vi "Apend Test Suite Result to Suites Element.vi"(8 "error in (no error)":errorcluster, 9 "Test Suite Result":T1, 10 "Test Suites Element in":refnum<k20>, 11 "XML Report In":refnum<class "XML Report.lvclass">) -> (0 "error out":errorcluster, 1 "Test Suite Element":refnum<k20>, 2 "Test Suites Element out":refnum<k20>, 3 "XML Report Out":refnum<class "XML Report.lvclass">)   [LabVIEW 2020, in "XML Report.lvclass"]
uses:
  XML Report.lvclass
  Result Types/Suite Results/Test Suite Result type.ctl
  Result Types/Assertion Result/Public/TypeDefs/Status.ctl
  Result Types/Case Result/Test Case Result type.ctl
  Result Types/Method Result/Method Result type.ctl
  Result Types/Assertion Result/Assertion Result type.ctl
  Result Types/Assertion Result/Public/TypeDefs/Assertion Type.ctl
  XML Report.lvclass/XML Report.ctl
  Result Types/Suite Results/Public/Count by Status.vi
  Result Types/Case Result/Public/Read Status.vi
  Result Types/Case Result/Private/Merge Status.vi
  Result Types/Method Result/Public/Read Status.vi
  <resource>/objmgr/DOMUserDefRef.rc
  Result Types/Suite Results/Test Suite Result.lvlib
  Result Types/Assertion Result/Assertion Result.lvlib
  Result Types/Method Result/Method Result.lvlib
  Result Types/Case Result/Test Case Result.lvlib
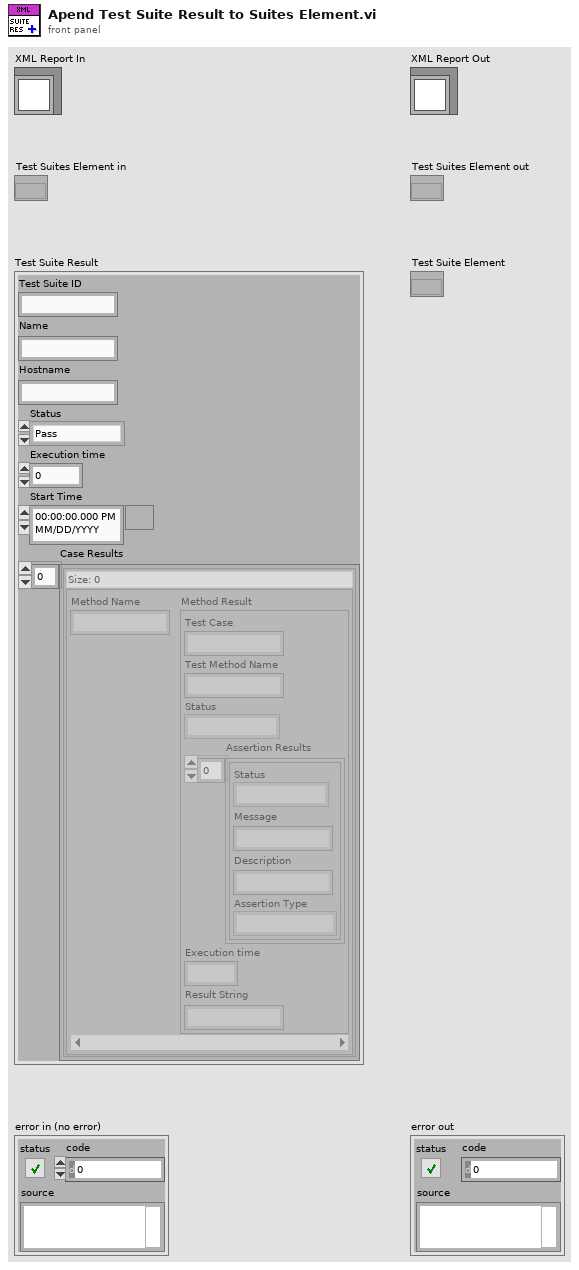
[diagram p1: front panel]
types:
  T1 = typedef "Test Suite Result.lvlib/Test Suite Result type.ctl" = cluster{"Test Suite ID":string, "Name":string, "Hostname":string, "Status":T2, "Execution time":dbl, "Start Time":timestamp, "Case Results":T3[]}
  T2 = typedef "Assertion Result.lvlib/Status.ctl" = enum16{"Pass", "Fail", "Error", "Skipped", "Setup Error", "Broken", "Teardown Error"}
  T3 = typedef "Test Case Result.lvlib/Test Case Result type.ctl" = map{string, T4}
  T4 = typedef "Method Result.lvlib/Method Result type.ctl" = cluster{"Test Case":string, "Test Method Name":string, "Status":T2, "Assertion Results":T5[], "Execution time":dbl, "Result String":string}
  T5 = typedef "Assertion Result.lvlib/Assertion Result type.ctl" = cluster{"Status":T2, "Message":string, "Description":string, "Assertion Type":T6}
  T6 = typedef "Assertion Result.lvlib/Assertion Type.ctl" = enum16{"None", "Pass", "Fail", "Skip", "Pass if Equal", "Fail if Equal", "Pass if Error", "Fail if Error", "Pass if", "Fail if"}
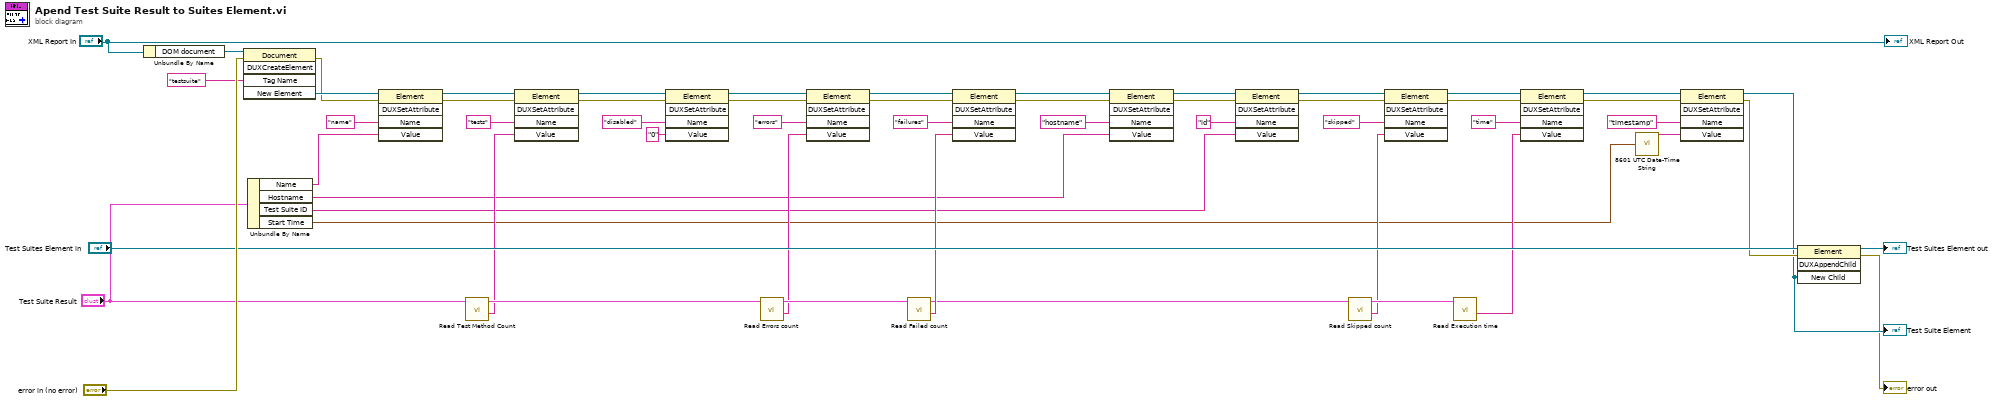
[diagram p0: block diagram]
diagram:
  n1 = Unbundle By Name("XML Report In") -> ("DOM document"=w53:refnum<k20>)
  n2 = invoke class="Document" method="DUXCreateElement"(reference=w53, error in="error in (no error)", "Tag Name"="testsuite") -> (error out=w16:errorcluster, "New Element"=w48:refnum<k20>)  [unwired: 2 in, 3 out]
  n3 = Unbundle By Name("Test Suite Result") -> ("Name"=w12:string, "Hostname"=w5:string, "Test Suite ID"=w4:string, "Start Time"=w2:timestamp)
  n4 = invoke class="Element" method="DUXSetAttribute"(reference=w48, error in=w16, "Name"="name", "Value"=w12) -> (reference out=w34:refnum<k20>, error out=w33:errorcluster)  [unwired: 1 in, 3 out]
  n5 = call "Read Test Method Count.vi"("Test Suite Result In"="Test Suite Result") -> ("Test Method count string"=w11:string, "Test Suite Result Out"=w37:T1)  [unwired: 8 in, 1 out]
  n6 = invoke class="Element" method="DUXSetAttribute"(reference=w34, error in=w33, "Name"="tests", "Value"=w11) -> (reference out=w32:refnum<k20>, error out=w31:errorcluster)  [unwired: 1 in, 3 out]
  n7 = invoke class="Element" method="DUXSetAttribute"(reference=w32, error in=w31, "Name"="disabled", "Value"="0") -> (reference out=w30:refnum<k20>, error out=w29:errorcluster)  [unwired: 1 in, 3 out]
  n8 = call "Read Errors count.vi"("Test Suite Result In"=w37) -> ("Error count string"=w10:string, "Test Suite Result Out"=w36:T1)  [unwired: 8 in, 1 out]
  n9 = invoke class="Element" method="DUXSetAttribute"(reference=w30, error in=w29, "Name"="errors", "Value"=w10) -> (reference out=w28:refnum<k20>, error out=w27:errorcluster)  [unwired: 1 in, 3 out]
  n10 = call "Read Failed count.vi"("Test Suite Result In"=w36) -> ("Failures count string"=w9:string, "Test Suite Result Out"=w3:T1)  [unwired: 8 in, 1 out]
  n11 = invoke class="Element" method="DUXSetAttribute"(reference=w28, error in=w27, "Name"="failures", "Value"=w9) -> (reference out=w26:refnum<k20>, error out=w25:errorcluster)  [unwired: 1 in, 3 out]
  n12 = invoke class="Element" method="DUXSetAttribute"(reference=w26, error in=w25, "Name"="hostname", "Value"=w5) -> (reference out=w24:refnum<k20>, error out=w23:errorcluster)  [unwired: 1 in, 3 out]
  n13 = invoke class="Element" method="DUXSetAttribute"(reference=w24, error in=w23, "Name"="id", "Value"=w4) -> (reference out=w22:refnum<k20>, error out=w21:errorcluster)  [unwired: 1 in, 3 out]
  n14 = call "Read Skipped count.vi"("Test Suite Result In"=w3) -> ("Skipped count string"=w8:string, "Test Suite Result Out"=w35:T1)  [unwired: 8 in, 1 out]
  n15 = invoke class="Element" method="DUXSetAttribute"(reference=w22, error in=w21, "Name"="skipped", "Value"=w8) -> (reference out=w20:refnum<k20>, error out=w19:errorcluster)  [unwired: 1 in, 3 out]
  n16 = call "Read Execution time.vi"("Test Suite Result In"=w35) -> ("Execution time string"=w7:string)  [unwired: 8 in, 2 out]
  n17 = invoke class="Element" method="DUXSetAttribute"(reference=w20, error in=w19, "Name"="time", "Value"=w7) -> (reference out=w18:refnum<k20>, error out=w17:errorcluster)  [unwired: 1 in, 3 out]
  n18 = call "8601 UTC Date-Time String.vi"("time stamp (Current Time)"=w2) -> ("8601 Date/Time String"=w6:string)  [unwired: 12 in, 2 out]
  n19 = invoke class="Element" method="DUXSetAttribute"(reference=w18, error in=w17, "Name"="timestamp", "Value"=w6) -> (reference out=w14:refnum<k20>, error out=w15:errorcluster)  [unwired: 1 in, 3 out]
  "Test Suite Element" <- w14
  n20 = invoke class="Element" method="DUXAppendChild"(reference="Test Suites Element in", error in=w15, "New Child"=w14) -> (reference out=→"Test Suites Element out":refnum<k20>, error out=→"error out":errorcluster)  [unwired: 1 in, 2 out]
  "XML Report Out" <- "XML Report In"
